vi "Shorten Directions.vi"(11 "Directions":T3[](array[typedef])) -> (3 "Direction with Distance":T1)   [LabVIEW 2019, in "Grassfire.lvclass"]
uses:
  Grassfire.lvclass
  Direction--enum.ctl
  Direction with distance--array.ctl
  Direction with distance--cluster.ctl
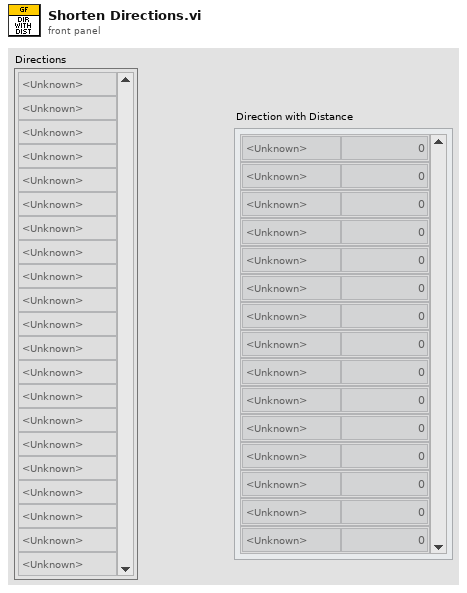
[diagram p1: front panel]
types:
  T1 = typedef "Grassfire.lvclass/Direction with distance--array.ctl" = T2[]
  T2 = typedef "Grassfire.lvclass/Direction with distance--cluster.ctl" = cluster{"Direction":T3, "Distance":i32}
  T3 = typedef "Grassfire.lvclass/Direction--enum.ctl" = enum16{"<Unknown>", "Right", "Down", "Left", "Up"}
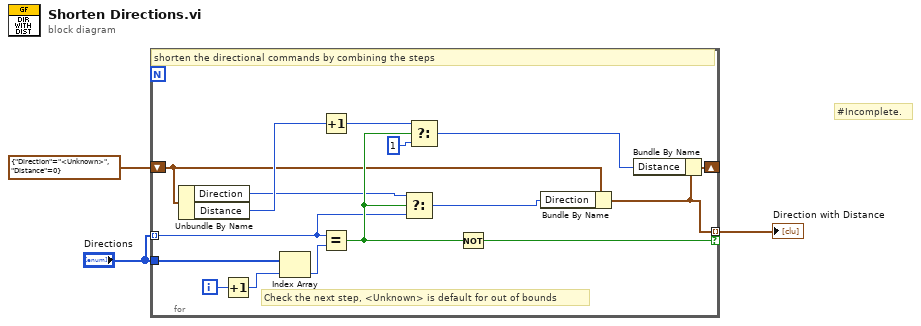
[diagram p0: block diagram]
diagram:
  # "#Incomplete."
  n1 = for {
    shift-right: [w13] -> _
    shift-left: T2 {"Direction"=enum."<Unknown>", "Distance"=0} ("Cluster") -> [w6]
    tunnel: "Directions" -> [w7] mode=indexing
    tunnel: [w4] -> w1 mode=indexing if=w10
    tunnel: "Directions" -> [w19]
    i -> [w18]
    # "Check the next step, <Unknown> is default for out of bounds"
    # "shorten the directional commands by combining the steps"
    n2 = Unbundle By Name(w6) -> ("Direction"=w8:T3, "Distance"=w14:i32)
    n3 = Increment(x=w18) -> (x+1=w17:i32)
    n4 = Index Array(array=w19, index=w17) -> (element=w16:T3)
    n5 = Increment(x=w14) -> (x+1=w15:i32)
    n6 = Equal?(x=w7, y=w16) -> (x = y?=w9:bool)
    n7 = Select(t=w8, s=w9, f=w7) -> (s? t:f=w5:T3)
    n8 = Select(t=w15, s=w9, f=1) -> (s? t:f=w11:i32)
    n9 = Not(x=w9) -> (.not. x?=w10:bool)
    n10 = Bundle By Name(cluster=w6, "Direction"=w5) -> (w4:T2)
    n11 = Bundle By Name(cluster=w4, "Distance"=w11) -> (w13:T2)
  }
  "Direction with Distance" <- w1
